vi "Main.vi"() -> ()   [LabVIEW 2021]
doc: "Use this template to build a simple state machine design pattern. Each state executes code and determines which state to transition to."
uses:
  controls/State.ctl
  controls/Data.ctl
  vmmso/vmmso.lvlib
panel:
  out "IO Read Return":u32 format="%x"
  out "IO4":bool
  out "IO0":bool
  out "Is IO Ready?":bool
  in  "DDS2 Amplitude":dbl=2000.0
  in  "DDS2 Bias":dbl
  in  "DDS2 Freq":dbl=1000.0
  in  "DDS2 Wave Style":u16(ring) items=["Sine", "Square", "Ramp"]
  in  "DDS1 Amplitude":dbl=2000.0
  in  "DDS1 Bias":dbl
  in  "DDS1 Freq":dbl=1000.0
  in  "DDS1 Wave Style":u16(ring) items=["Sine", "Square", "Ramp"]
  out "Is Data Ready？":bool
  out "ReadVoltageData Return":u32
  out "Voltage Wave":dbl[][](graph)
  out "Capture Return":i32
  out "Device is OK?":bool
  out "Support Samples":u32[](array[numeric])
  in  "Exit":bool
  # "DDS1"
  # "DDS2"
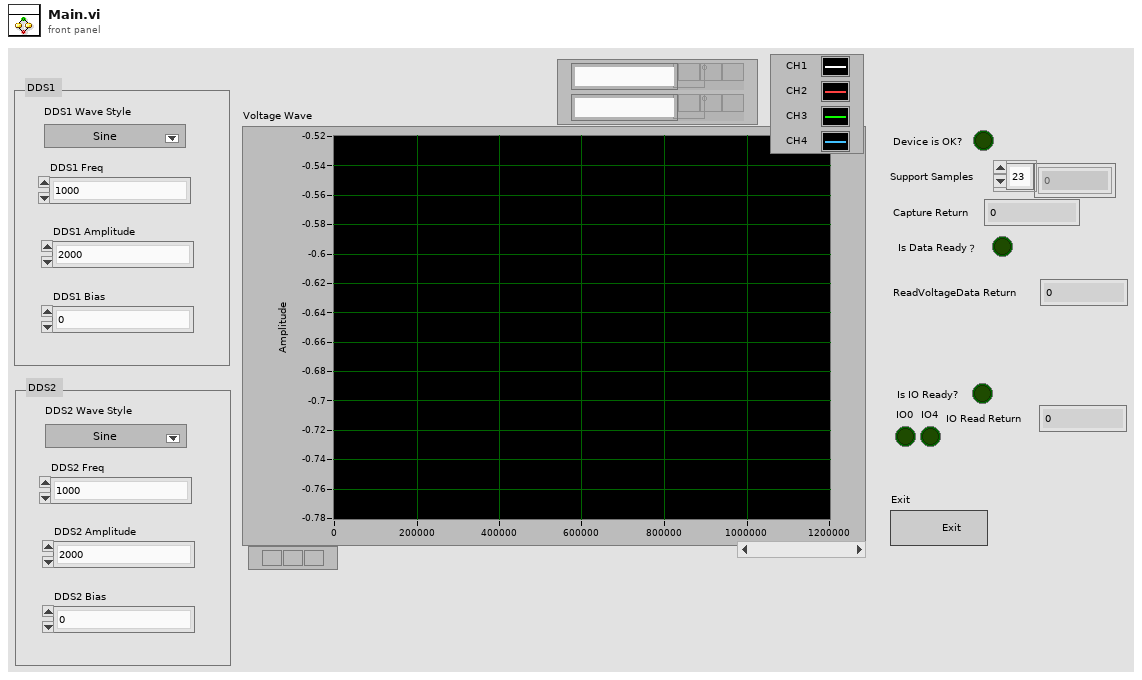
[diagram p1: front panel]
types:
  T1 = typedef "Data.ctl" = cluster{"Boolean <Is Exit>":bool, "String <Replace Me>":string, "Numeric <Replace Me>":dbl}
  T2 = typedef "State.ctl" = enum16{"Initialize", "Wait for UsbIn", "Init Osc and Dds", "Wait for Event", "Capture", "Read Voltage", "Read IO", "Exit"}
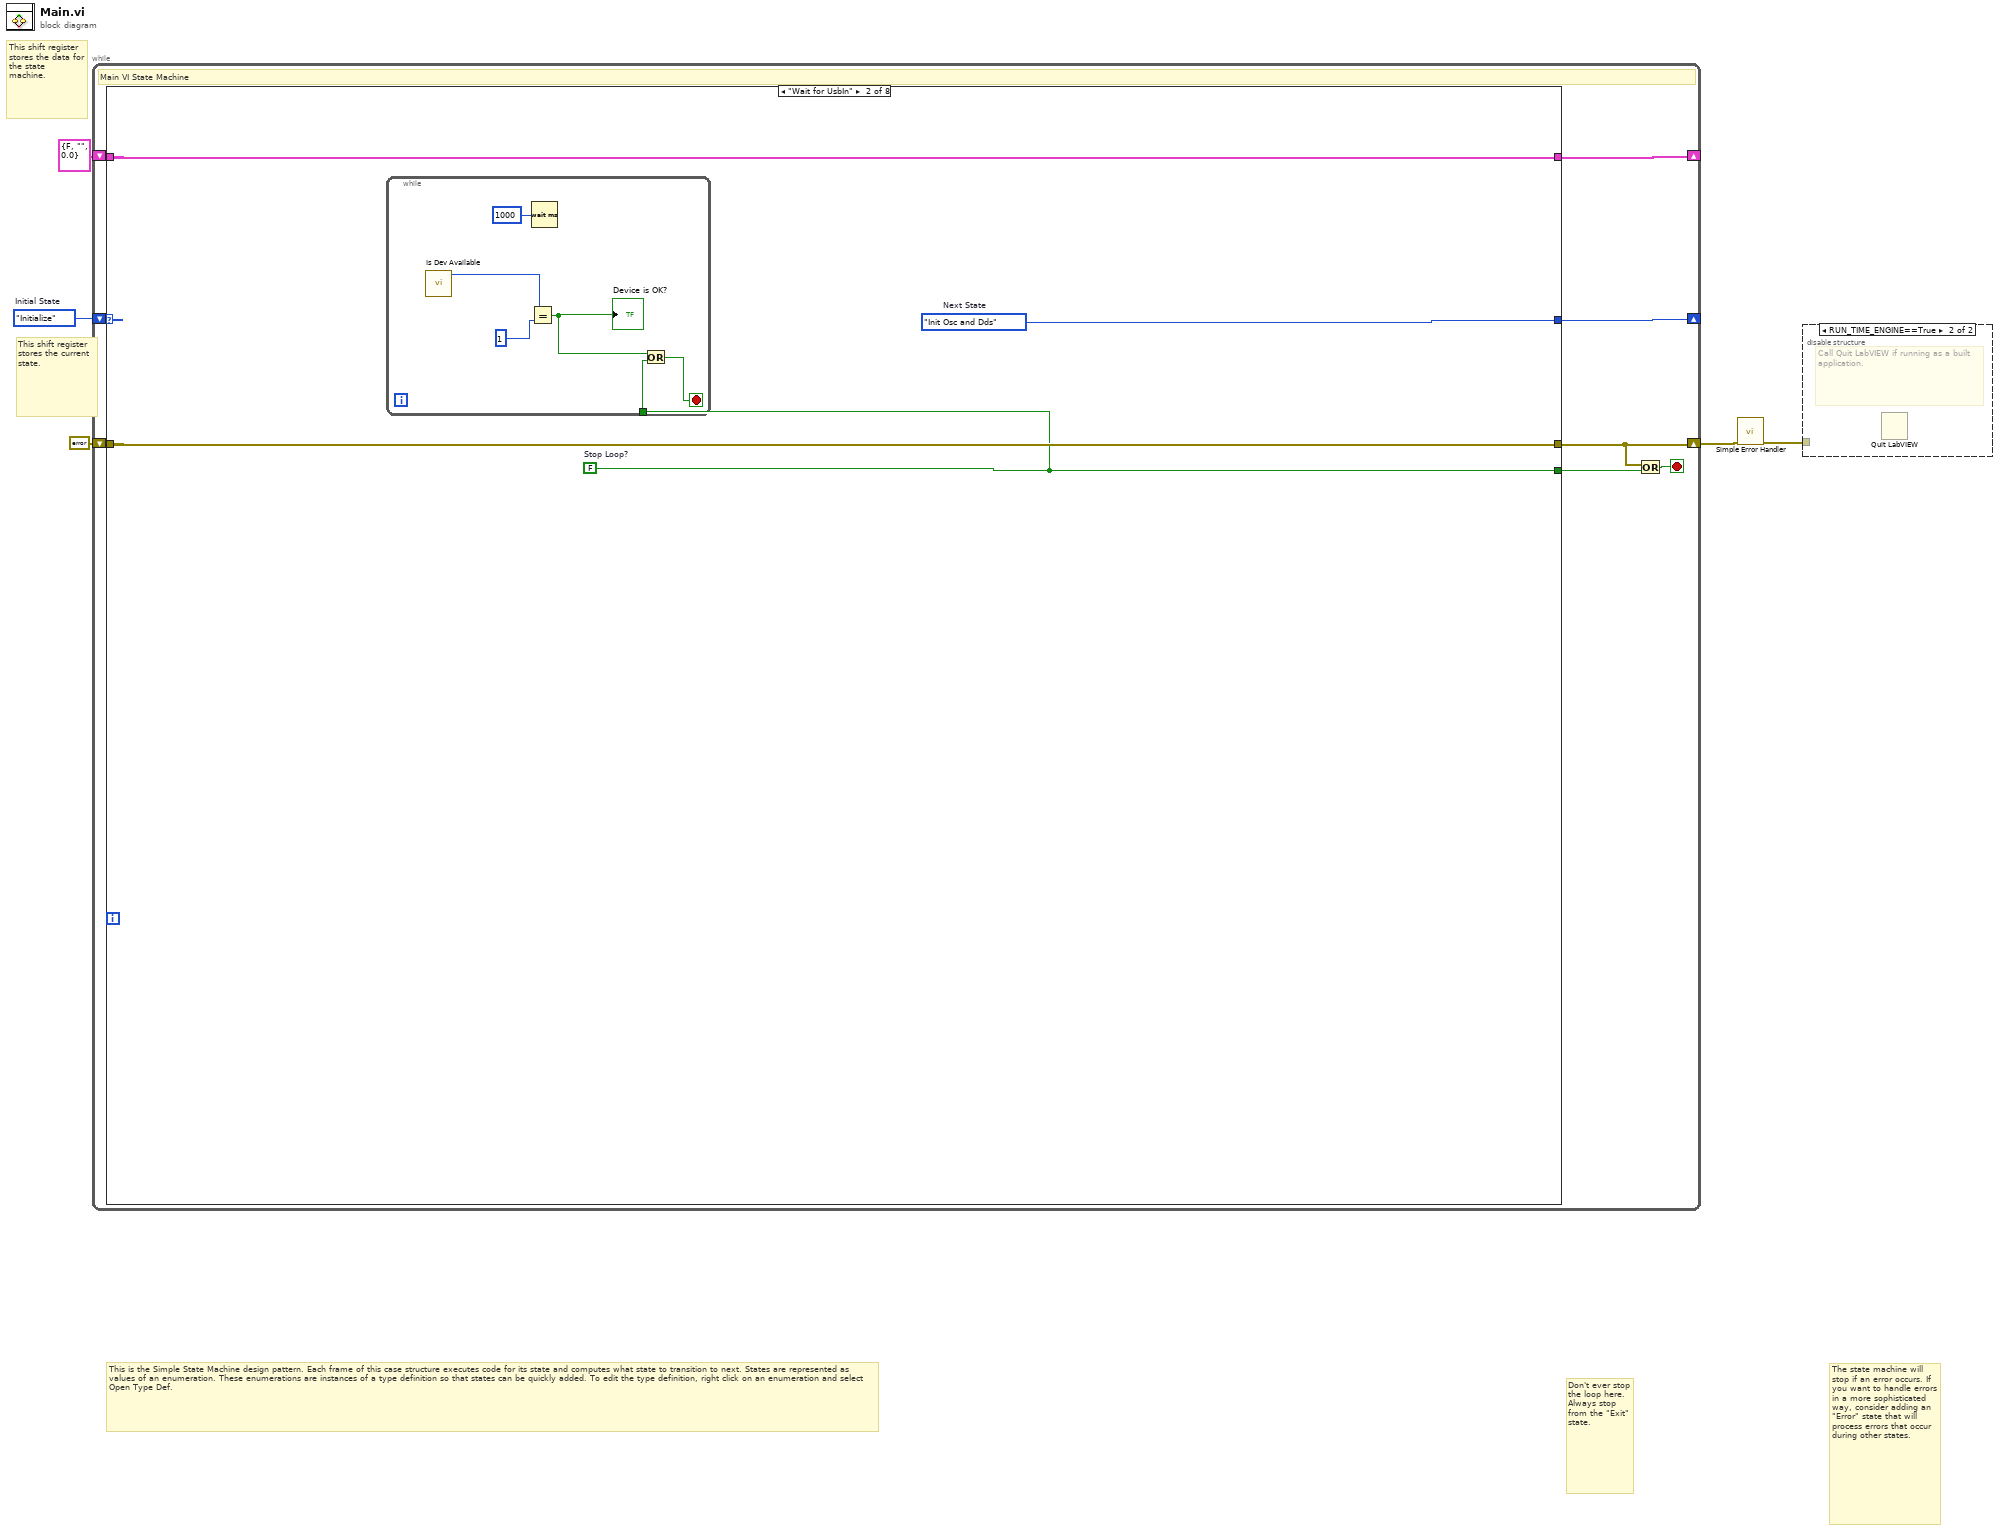
[diagram p0: block diagram]
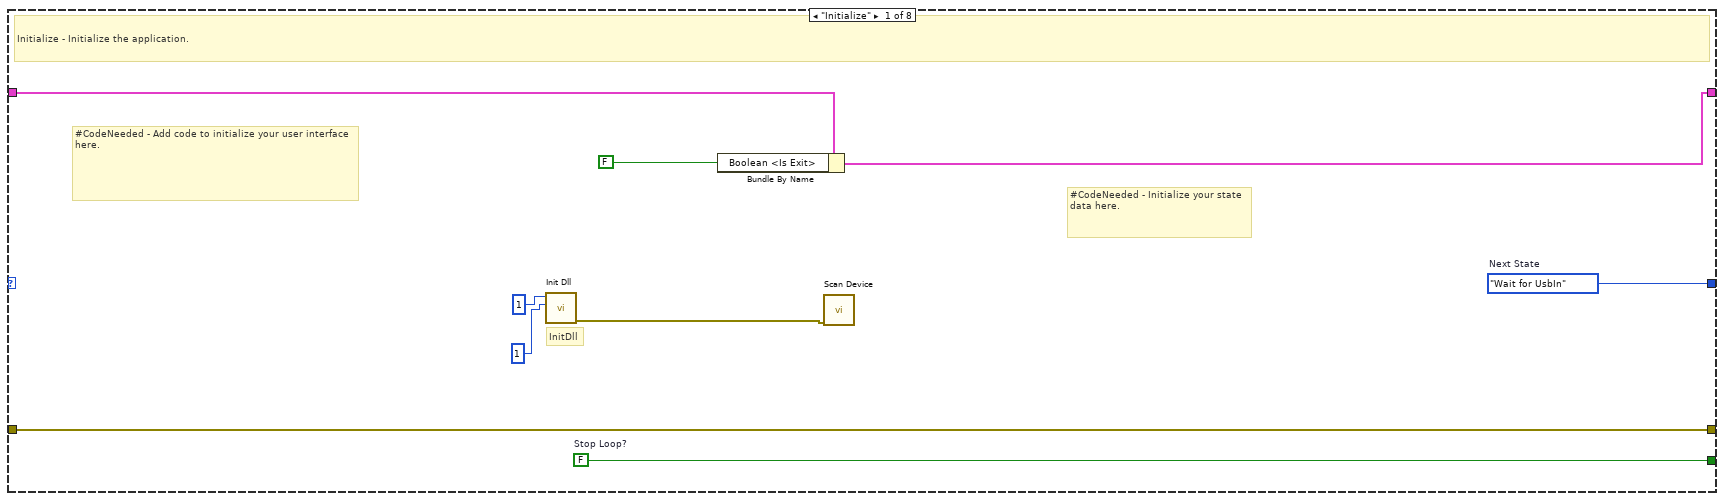
[diagram p3: hidden frame]
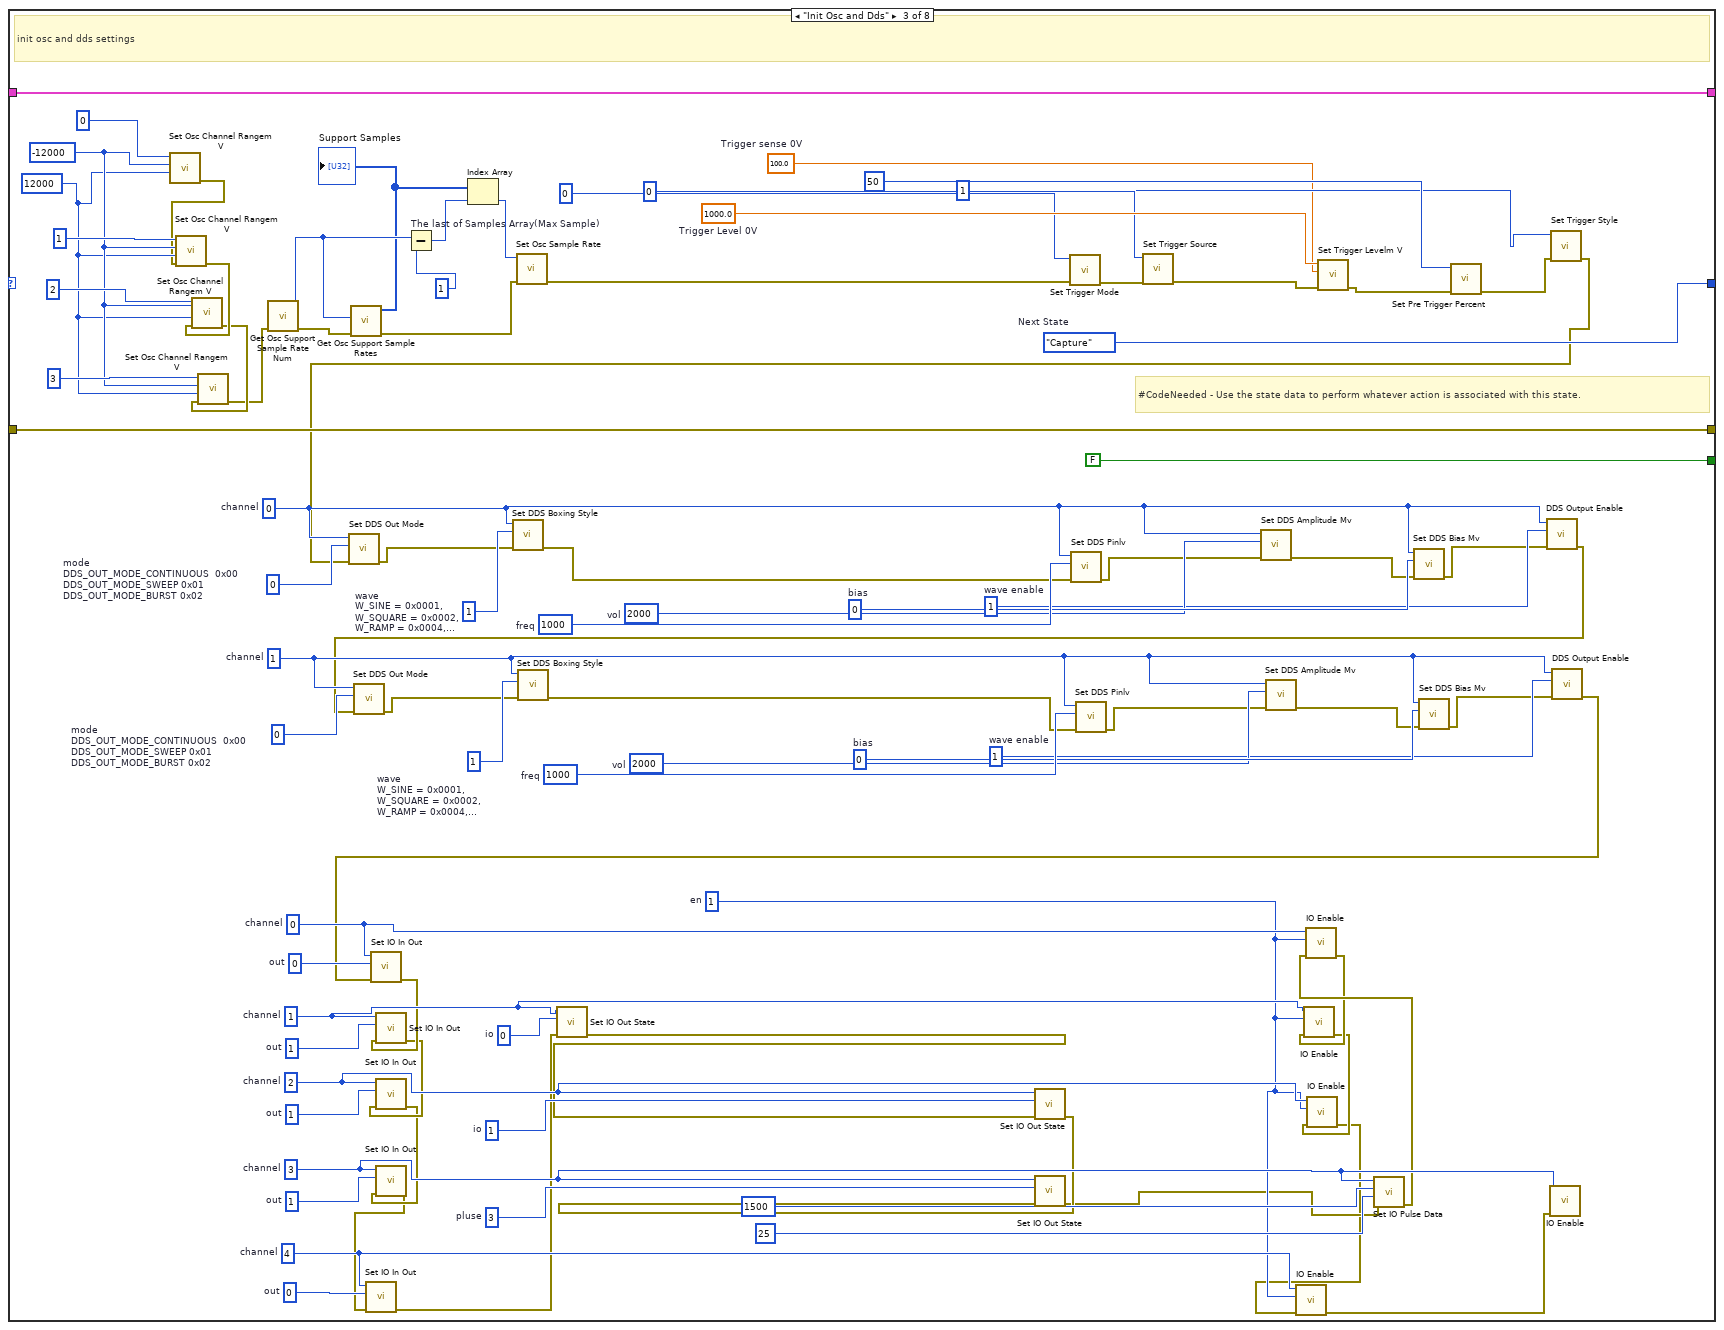
[diagram p4: hidden frame]
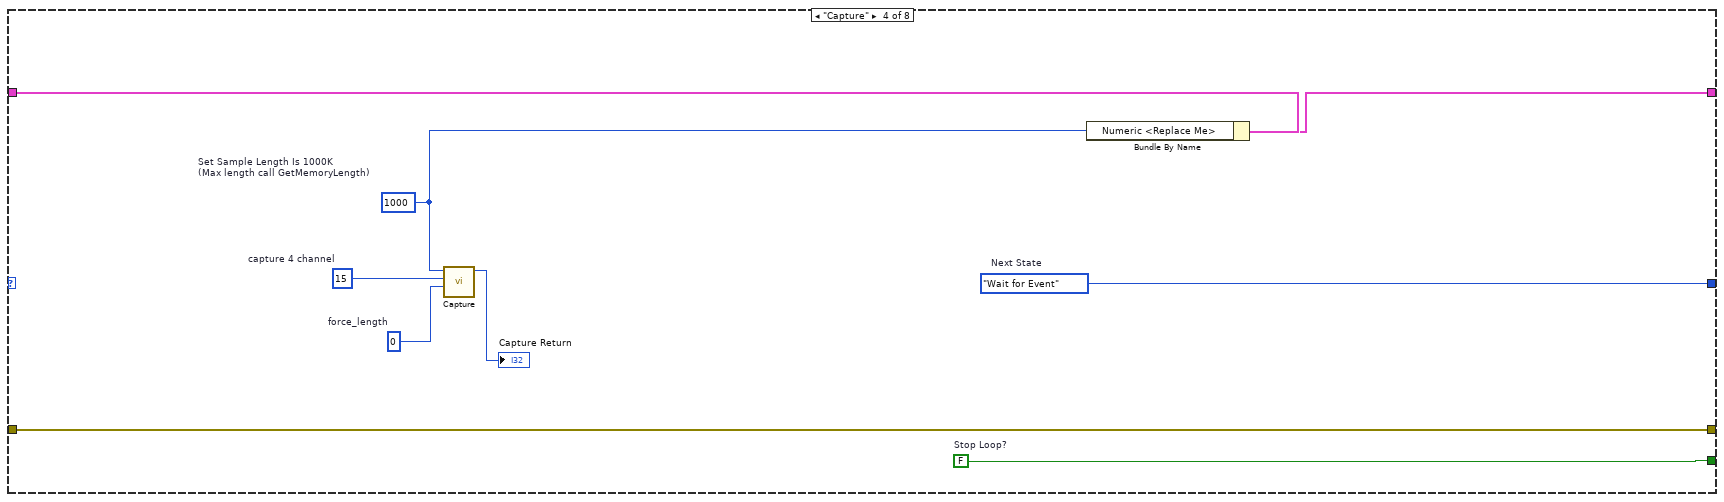
[diagram p5: hidden frame]
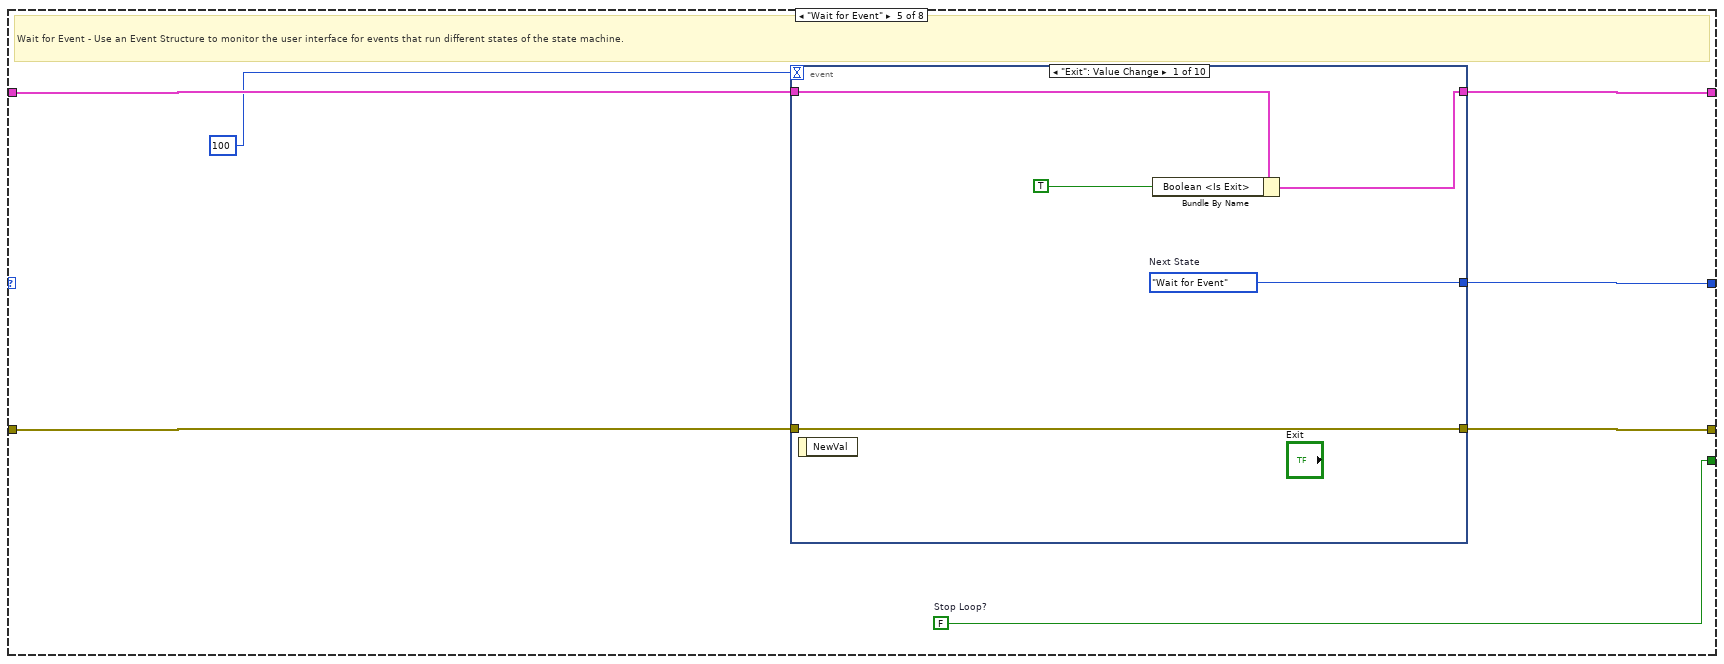
[diagram p6: hidden frame]
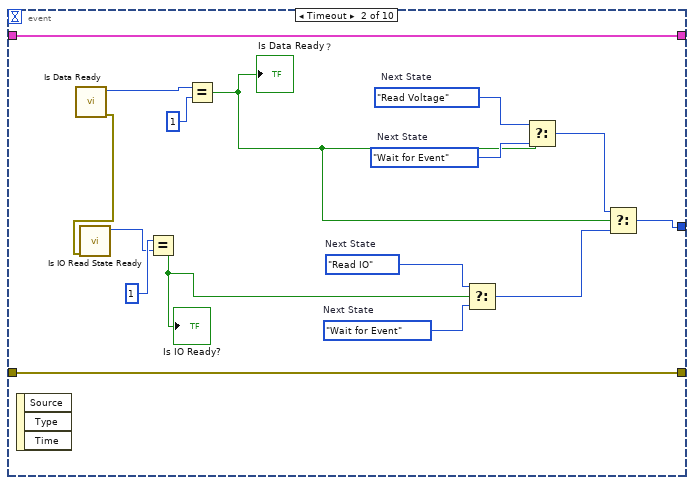
[diagram p7: hidden frame]
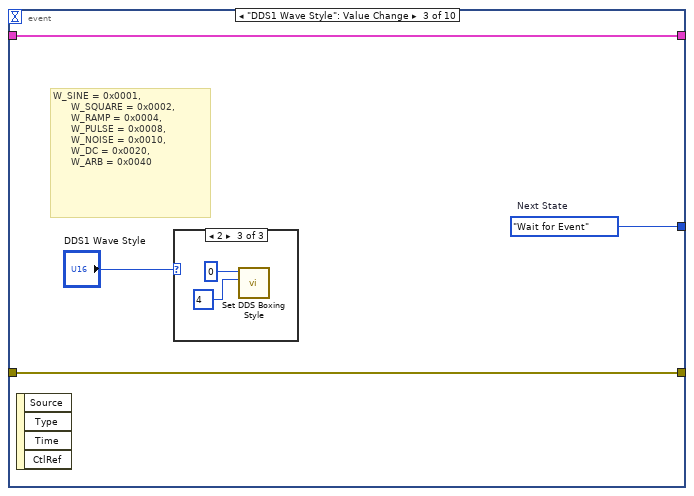
[diagram p8: hidden frame]
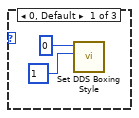
[diagram p9: hidden frame]
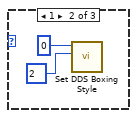
[diagram p10: hidden frame]
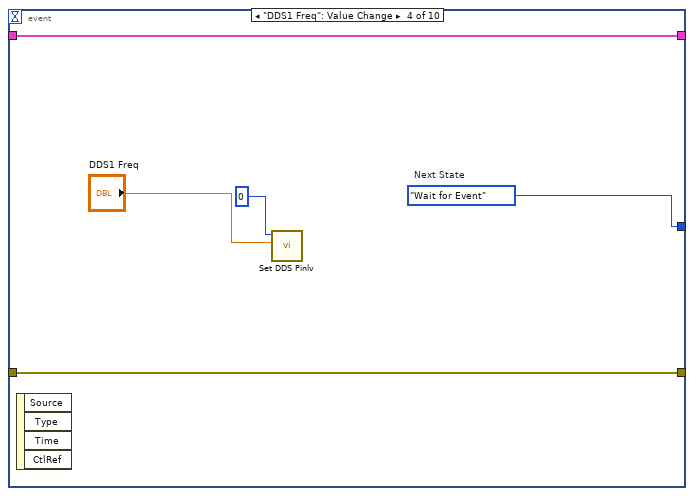
[diagram p11: hidden frame]
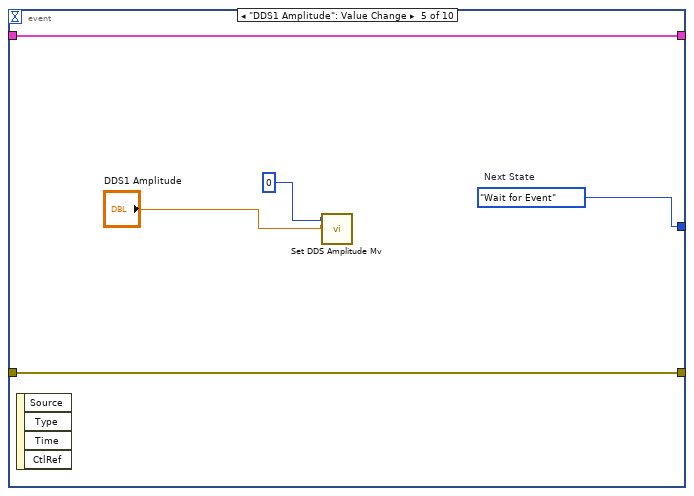
[diagram p12: hidden frame]
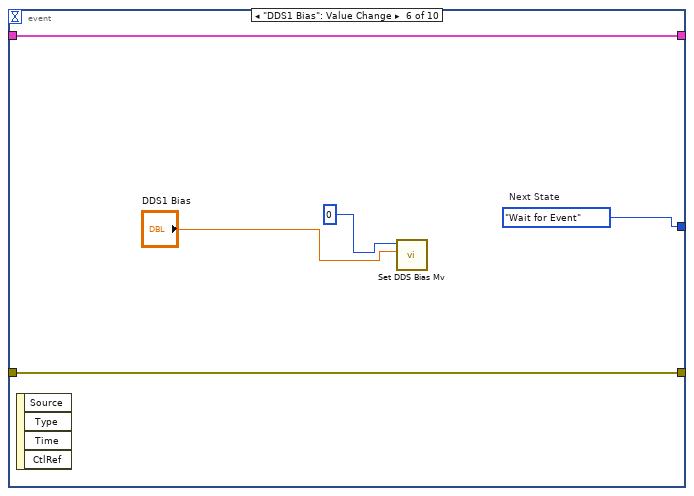
[diagram p13: hidden frame]
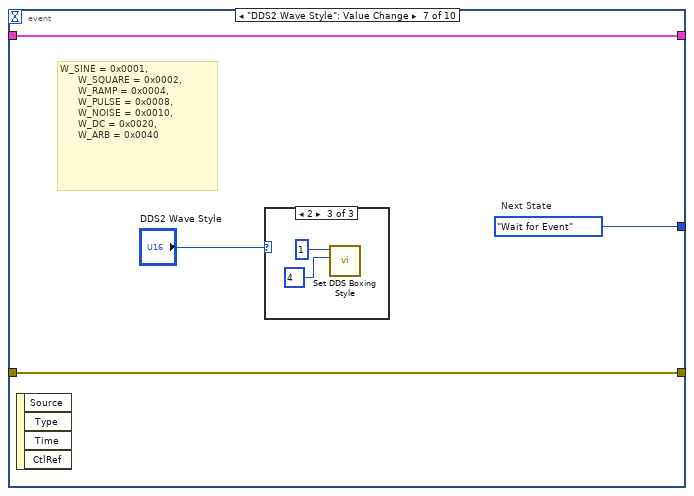
[diagram p14: hidden frame]
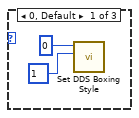
[diagram p15: hidden frame]
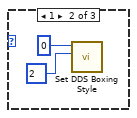
[diagram p16: hidden frame]
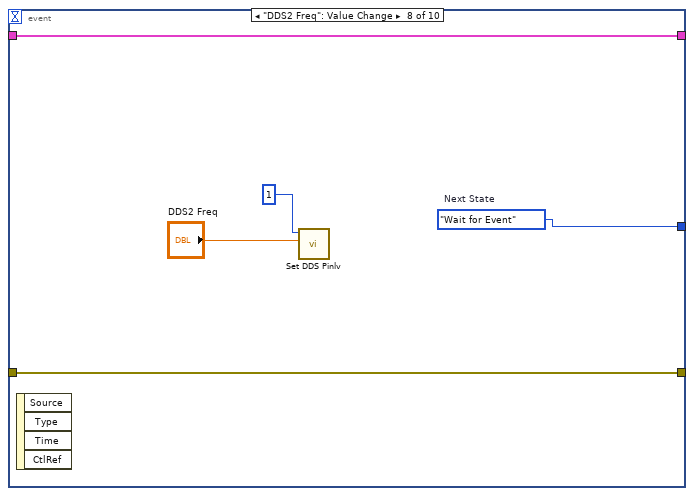
[diagram p17: hidden frame]
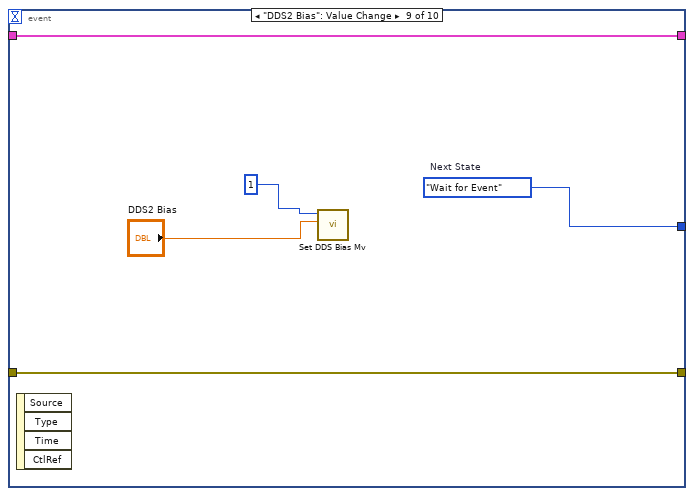
[diagram p18: hidden frame]
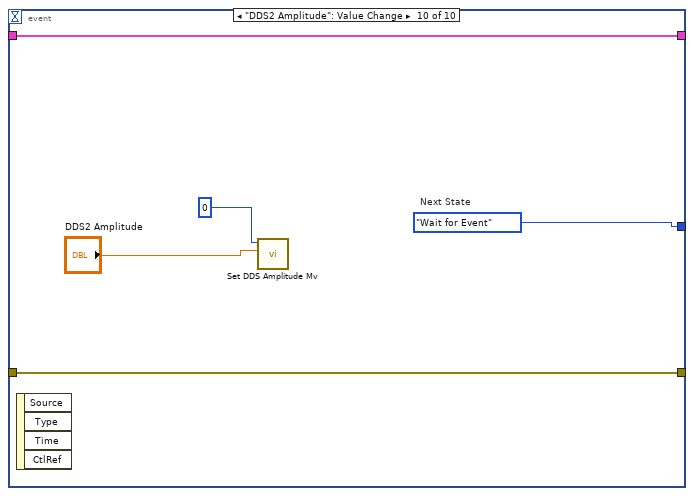
[diagram p19: hidden frame]
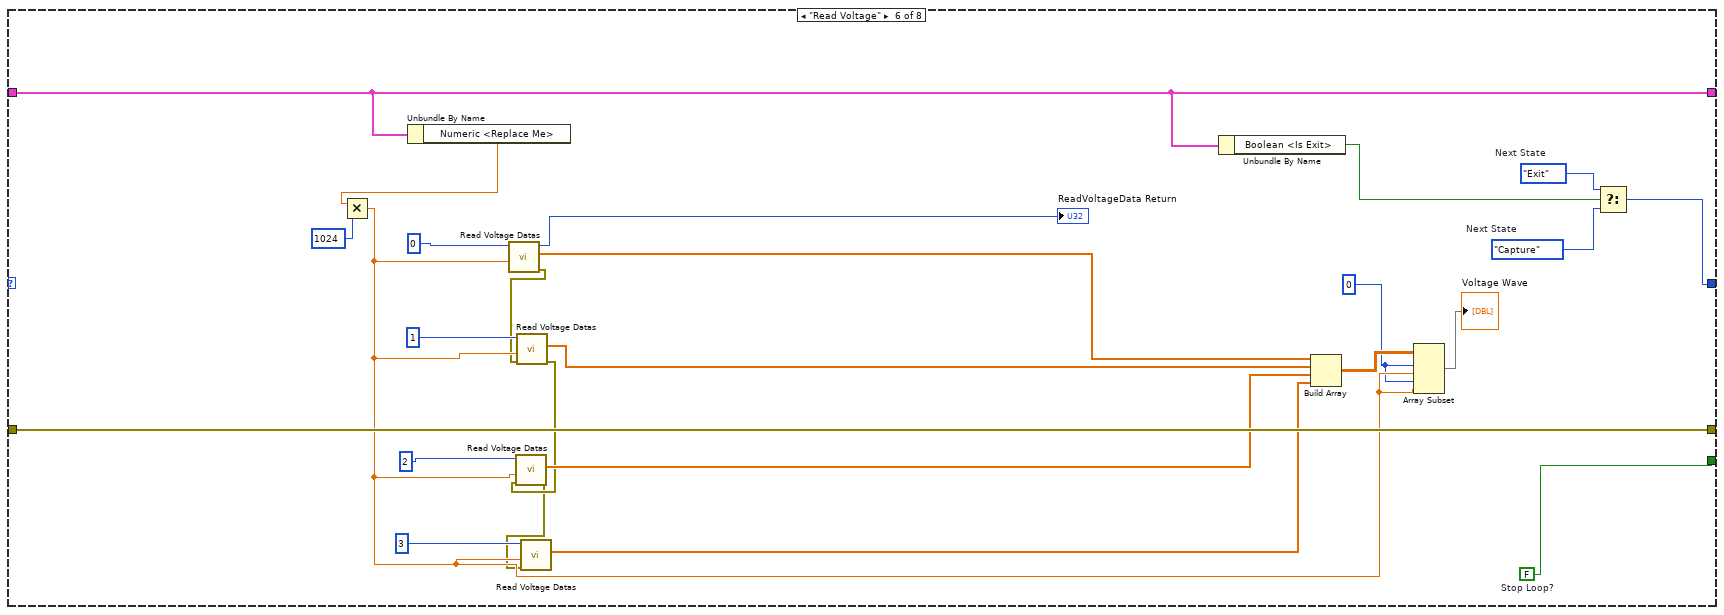
[diagram p20: hidden frame]
diagram:
  w5 = State."Initialize"  # Initial State
  # "Don't ever stop the loop here. Always stop from the \"Exit\" state."
  # "The state machine will stop if an error occurs. If you want to handle errors in a more sophisticated way, consider adding an \"Error\" state that will process errors that occur during other states."
  # "This shift register stores the data for the state machine."
  # "This is the Simple State Machine design pattern. Each frame of this case structure executes code for its state and computes what state to transition to next. States are represented as values of an enumeration. These enumerations are instances of a type definition so that states can be quickly added. To edit the type definition, right click on an enumeration and select Open Type Def."
  # "This shift register stores the current state."
  n1 = while {
    shift-right: [w12] -> _
    shift-left: w5 -> [w13]
    shift-right: [w10] -> _
    shift-left: T1 {"Boolean <Is Exit>"=FALSE, "String <Replace Me>"="", "Numeric <Replace Me>"=0.0} ("Data") -> [w11]
    shift-right: [w7] -> w2
    shift-left: errorcluster {"status"=FALSE, "code"=0, "source"=""} ("error constant") -> [w9]
    stop <- w8 stop-if-true
    # "Main VI State Machine"
    n2 = case shown="\"Wait for UsbIn\"" w13 {
      tunnel: [w22 w25 w120 w128 w136 w209 w234 w248] -> w12
      tunnel: w11 -> [w15 w23 w118 w123 w135 w212 w243 w247]
      tunnel: [w14 w23 w118 w122 w134 w212 w243 w247] -> w10
      tunnel: w9 -> [w20 w26 w117 w129 w133 w232 w242 w245]
      tunnel: [w20 w26 w117 w129 w132 w232 w242 w245] -> w7
      tunnel: [w21 w24 FALSE ("Stop Loop?") w127 w130 w231 w233 w246] -> w6
      frame "Initialize" {
        w21 = FALSE  # Stop Loop?
        w22 = State."Wait for UsbIn"  # Next State
        # "InitDll"
        # "#CodeNeeded - Initialize your state data here."
        # "#CodeNeeded - Add code to initialize your user interface here."
        # "Initialize - Initialize the application."
        n3 = call "Init Dll.vi"("en_hard_watchdog"=1 ("channel"), "en_log"=1 ("channel")) -> ("error out"=w17:errorcluster)  [unwired: 8 in, 1 out]
        n4 = Bundle By Name(cluster=w15, "Boolean <Is Exit>"=FALSE) -> (w14:T1)
        n5 = call "Scan Device.vi"("error in (no error)"=w17) -> ()  [unwired: 9 in, 2 out]
      }
      frame "Wait for UsbIn" {
        w25 = State."Init Osc and Dds"  # Next State
        w24 = FALSE  # Stop Loop?
        n6 = while {
          tunnel: w24 -> [w30]
          stop <- w29 stop-if-true
          n7 = call "Is Dev Available.vi"() -> ("function return"=w28:i32)  [unwired: 10 in, 1 out]
          n8 = Equal?(x=w28, y=1 ("channel")) -> (x = y?=w27:bool)
          "Device is OK?" <- w27
          n9 = Wait (ms)(milliseconds to wait=u32 1000 ("等待时间（毫秒）")) -> ()  [unwired: 1 out]
          n10 = Or(x=w27, y=w30) -> (x .or. y?=w29:bool)
        }
      }
      frame "Init Osc and Dds" {
        w72 = i8 0  # out
        w71 = i8 4  # channel
        w76 = i8 3  # pluse
        w77 = i8 1  # out
        w75 = i8 3  # channel
        w70 = i8 1  # en
        w81 = i8 0  # io
        w82 = i8 1  # io
        w83 = i8 1  # out
        w78 = i8 2  # channel
        w84 = i8 1  # out
        w79 = i8 1  # channel
        w85 = i8 0  # out
        w80 = i8 0  # channel
        w86 = sgl 100.0  # Trigger sense 0V
        w93 = i8 0  # mode DDS_OUT_MODE_CONTINUOUS  0x00 DDS_OUT_MODE_SWEEP 0x01 DDS_OUT_MODE_BURST 0x02
        w95 = i8 1  # wave enable
        w97 = u32 0  # bias
        w96 = u32 2000  # vol
        w98 = u32 1000  # freq
        w99 = i8 1  # wave  W_SINE = 0x0001,  W_SQUARE = 0x0002,  W_RAMP = 0x0004,  W_PULSE = 0x0008,  W_NOISE = 0x0010,  W_DC = 0x0020,  W_ARB = 0x0040
        w94 = i8 1  # channel
        w100 = i8 0  # mode DDS_OUT_MODE_CONTINUOUS  0x00 DDS_OUT_MODE_SWEEP 0x01 DDS_OUT_MODE_BURST 0x02
        w102 = i8 1  # wave enable
        w104 = u32 0  # bias
        w103 = u32 2000  # vol
        w105 = u32 1000  # freq
        w106 = i8 1  # wave  W_SINE = 0x0001,  W_SQUARE = 0x0002,  W_RAMP = 0x0004,  W_PULSE = 0x0008,  W_NOISE = 0x0010,  W_DC = 0x0020,  W_ARB = 0x0040
        w101 = i8 0  # channel
        w114 = sgl 1000.0  # Trigger Level 0V
        w88 = 12000 ("minmv")
        w89 = -12000 ("minmv")
        w120 = State."Capture"  # Next State
        # "#CodeNeeded - Use the state data to perform whatever action is associated with this state."
        # "init osc and dds settings"
        n11 = call "Set Osc Channel Rangem V.vi"("maxmv"=w88, "minmv"=w89, "channel"=0) -> ("error out"=w69:errorcluster)  [unwired: 7 in, 1 out]
        n12 = call "Set Osc Channel Rangem V.vi"("error in (no error)"=w69, "maxmv"=w88, "minmv"=w89, "channel"=1) -> ("error out"=w68:errorcluster)  [unwired: 6 in, 1 out]
        n13 = call "Set Osc Channel Rangem V.vi"("error in (no error)"=w68, "maxmv"=w88, "minmv"=w89, "channel"=2) -> ("error out"=w67:errorcluster)  [unwired: 6 in, 1 out]
        n14 = call "Set Osc Channel Rangem V.vi"("error in (no error)"=w67, "maxmv"=w88, "minmv"=w89, "channel"=3) -> ("error out"=w66:errorcluster)  [unwired: 6 in, 1 out]
        n15 = call "Get Osc Support Sample Rate Num.vi"("error in (no error)"=w66) -> ("error out"=w65:errorcluster, "function return"=w111:i32)  [unwired: 9 in]
        n16 = call "Get Osc Support Sample Rates.vi"("error in (no error)"=w65, "maxnum"=w111) -> ("error out"=w64:errorcluster, "sample out"=w108:u32[])  [unwired: 7 in, 1 out]
        "Support Samples" <- w108
        n17 = Subtract "The last of Samples Array(Max Sample)"(x=w111, y=1 ("front")) -> (x-y=w113:i32)
        n18 = Index Array(array=w108, index=w113) -> (element=w87:u32)
        n19 = call "Set Osc Sample Rate.vi"("error in (no error)"=w64, "sample"=w87) -> ("error out"=w63:errorcluster)  [unwired: 8 in, 1 out]
        n20 = call "Set Trigger Mode.vi"("error in (no error)"=w63, "mode"=0 ("front")) -> ("error out"=w62:errorcluster)  [unwired: 9 in]
        n21 = call "Set Trigger Source.vi"("error in (no error)"=w62, "source"=0 ("front")) -> ("error out"=w61:errorcluster)  [unwired: 9 in]
        n22 = call "Set Trigger Levelm V.vi"("error in (no error)"=w61, "sense_mv"=w86, "level_mv"=w114) -> ("error out"=w60:errorcluster)  [unwired: 8 in]
        n23 = call "Set Pre Trigger Percent.vi"("error in (no error)"=w60, "front"=50) -> ("error out"=w59:errorcluster)  [unwired: 9 in]
        n24 = call "Set Trigger Style.vi"("error in (no error)"=w59, "style"=u32 1) -> ("error out"=w58:errorcluster)  [unwired: 9 in]
        n25 = call "Set DDS Out Mode.vi"("error in (no error)"=w58, "out_mode"=w100, "channel_index"=w101) -> ("error out"=w57:errorcluster)  [unwired: 8 in]
        n26 = call "Set DDS Boxing Style.vi"("error in (no error)"=w57, "boxing"=w106, "channel_index"=w101) -> ("error out"=w56:errorcluster)  [unwired: 8 in]
        n27 = call "Set DDS Pinlv.vi"("error in (no error)"=w56, "pinlv"=w105, "channel_index"=w101) -> ("error out"=w55:errorcluster)  [unwired: 8 in]
        n28 = call "Set DDS Amplitude Mv.vi"("error in (no error)"=w55, "amplitdude"=w103, "channel_index"=w101) -> ("error out"=w54:errorcluster)  [unwired: 8 in]
        n29 = call "Set DDS Bias Mv.vi"("error in (no error)"=w54, "bias"=w104, "channel_index"=w101) -> ("error out"=w53:errorcluster)  [unwired: 8 in]
        n30 = call "DDS Output Enable.vi"("error in (no error)"=w53, "enable"=w102, "channel_index"=w101) -> ("error out"=w52:errorcluster)  [unwired: 8 in]
        n31 = call "Set DDS Out Mode.vi"("error in (no error)"=w52, "out_mode"=w93, "channel_index"=w94) -> ("error out"=w51:errorcluster)  [unwired: 8 in]
        n32 = call "Set DDS Boxing Style.vi"("error in (no error)"=w51, "boxing"=w99, "channel_index"=w94) -> ("error out"=w50:errorcluster)  [unwired: 8 in]
        n33 = call "Set DDS Pinlv.vi"("error in (no error)"=w50, "pinlv"=w98, "channel_index"=w94) -> ("error out"=w49:errorcluster)  [unwired: 8 in]
        n34 = call "Set DDS Amplitude Mv.vi"("error in (no error)"=w49, "amplitdude"=w96, "channel_index"=w94) -> ("error out"=w48:errorcluster)  [unwired: 8 in]
        n35 = call "Set DDS Bias Mv.vi"("error in (no error)"=w48, "bias"=w97, "channel_index"=w94) -> ("error out"=w47:errorcluster)  [unwired: 8 in]
        n36 = call "DDS Output Enable.vi"("error in (no error)"=w47, "enable"=w95, "channel_index"=w94) -> ("error out"=w46:errorcluster)  [unwired: 8 in]
        n37 = call "Set IO In Out.vi"("error in (no error)"=w46, "inout"=w85, "channel"=w80) -> ("error out"=w45:errorcluster)  [unwired: 8 in]
        n38 = call "Set IO In Out.vi"("error in (no error)"=w45, "inout"=w84, "channel"=w79) -> ("error out"=w44:errorcluster)  [unwired: 8 in]
        n39 = call "Set IO In Out.vi"("error in (no error)"=w44, "inout"=w83, "channel"=w78) -> ("error out"=w43:errorcluster)  [unwired: 8 in]
        n40 = call "Set IO In Out.vi"("error in (no error)"=w43, "inout"=w77, "channel"=w75) -> ("error out"=w42:errorcluster)  [unwired: 8 in]
        n41 = call "Set IO In Out.vi"("error in (no error)"=w42, "inout"=w72, "channel"=w71) -> ("error out"=w41:errorcluster)  [unwired: 8 in]
        n42 = call "Set IO Out State.vi"("error in (no error)"=w41, "state"=w81, "channel"=w79) -> ("error out"=w40:errorcluster)  [unwired: 8 in]
        n43 = call "Set IO Out State.vi"("error in (no error)"=w40, "state"=w82, "channel"=w78) -> ("error out"=w39:errorcluster)  [unwired: 8 in]
        n44 = call "Set IO Out State.vi"("error in (no error)"=w39, "state"=w76, "channel"=w75) -> ("error out"=w38:errorcluster)  [unwired: 8 in]
        n45 = call "Set IO Pulse Data.vi"("error in (no error)"=w38, "duty"=25 ("minmv"), "hz"=1500 ("minmv"), "channel"=w75) -> ("error out"=w37:errorcluster)  [unwired: 7 in]
        n46 = call "IO Enable.vi"("error in (no error)"=w37, "enable"=w70, "channel"=w80) -> ("error out"=w36:errorcluster)  [unwired: 8 in]
        n47 = call "IO Enable.vi"("error in (no error)"=w36, "enable"=w70, "channel"=w79) -> ("error out"=w35:errorcluster)  [unwired: 8 in]
        n48 = call "IO Enable.vi"("error in (no error)"=w35, "enable"=w70, "channel"=w78) -> ("error out"=w34:errorcluster)  [unwired: 8 in]
        n49 = call "IO Enable.vi"("error in (no error)"=w34, "enable"=w70, "channel"=w71) -> ("error out"=w33:errorcluster)  [unwired: 8 in]
        n50 = call "IO Enable.vi"("error in (no error)"=w33, "channel"=w75) -> ()  [unwired: 9 in, 1 out]
      }
      frame "Capture" {
        w124 = i8 0  # force_length
        w121 = u32 1000  # Set Sample Length Is 1000K (Max length call GetMemoryLength)
        w125 = i8 15  # capture 4 channel
        w127 = FALSE  # Stop Loop?
        w128 = State."Wait for Event"  # Next State
        n51 = call "Capture.vi"("force_length"=w124, "capture_channel"=w125, "length"=w121) -> ("function return"=→"Capture Return":i32)  [unwired: 7 in, 1 out]
        n52 = Bundle By Name(cluster=w123, "Numeric <Replace Me>"=w121) -> (w122:T1)
      }
      frame "Wait for Event" {
        w130 = FALSE  # Stop Loop?
        # "Wait for Event - Use an Event Structure to monitor the user interface for events that run different states of the state machine."
        n53 = event shown="[0] \"Exit\": Value Change" {
          selector: _ -> [_ _ _ _ _ _ _ _ _ _]
          dyn-events: _ -> [_ _ _ _ _ _ _ _ _ _]
          timeout: 100 ("y") -> [_ _ _ _ _ _ _ _ _ _]
          tunnel: [w141 w144 w158 w170 w175 w180 w184 w194 w199 w204] -> w136
          tunnel: w135 -> [w138 w157 w161 w172 w177 w182 w186 w197 w202 w207]
          tunnel: [w137 w157 w161 w172 w177 w182 w186 w197 w202 w207] -> w134
          tunnel: w133 -> [w140 w156 w160 w171 w176 w181 w185 w196 w201 w206]
          tunnel: [w140 w156 w160 w171 w176 w181 w185 w196 w201 w206] -> w132
          event "Exit": Value Change {
            w141 = State."Wait for Event"  # Next State
            n54 = event-data() -> ()  [unwired: 1 in, 1 out]
            n55 = Bundle By Name(cluster=w138, "Boolean <Is Exit>"=TRUE) -> (w137:T1)
          }
          event Timeout {
            w149 = State."Wait for Event"  # Next State
            w150 = State."Read IO"  # Next State
            w152 = State."Wait for Event"  # Next State
            w153 = State."Read Voltage"  # Next State
            n56 = event-data() -> ()  [unwired: 1 in, 3 out]
            n57 = call "Is Data Ready.vi"() -> ("error out"=w142:errorcluster, "function return"=w155:i32)  [unwired: 10 in]
            n58 = call "Is IO Read State Ready.vi"("error in (no error)"=w142) -> ("function return"=w143:i32)  [unwired: 9 in, 1 out]
            n59 = Equal?(x=1 ("y"), y=w143) -> (x = y?=w151:bool)
            "Is IO Ready?" <- w151
            n60 = Equal?(x=w155, y=1) -> (x = y?=w145:bool)
            "Is Data Ready？" <- w145
            n61 = Select(t=w150, s=w151, f=w149) -> (s? t:f=w147:T2)
            n62 = Select(t=w153, s=w145, f=w152) -> (s? t:f=w146:T2)
            n63 = Select(t=w146, s=w145, f=w147) -> (s? t:f=w144:T2)
          }
          event "DDS1 Wave Style": Value Change {
            w158 = State."Wait for Event"  # Next State
            # "W_SINE = 0x0001, \n\t\t\t\t\t\tW_SQUARE = 0x0002, \n\t\t\t\t\t\tW_RAMP = 0x0004, \n\t\t\t\t\t\tW_PULSE = 0x0008, \n\t\t\t\t\t\tW_NOISE = 0x0010, \n\t\t\t\t\t\tW_DC = 0x0020, \n\t\t\t\t\t\tW_ARB = 0x0040"
            n64 = event-data() -> ()  [unwired: 1 in, 4 out]
            n65 = case shown="2" "DDS1 Wave Style" {
              frame 0, Default {
                n66 = call "Set DDS Boxing Style.vi"("boxing"=1 ("y"), "channel_index"=0 ("y")) -> ()  [unwired: 9 in, 1 out]
              }
              frame 1 {
                n67 = call "Set DDS Boxing Style.vi"("boxing"=2 ("y"), "channel_index"=0 ("y")) -> ()  [unwired: 9 in, 1 out]
              }
              frame 2 {
                n68 = call "Set DDS Boxing Style.vi"("boxing"=4 ("y"), "channel_index"=0 ("y")) -> ()  [unwired: 9 in, 1 out]
              }
            }
          }
          event "DDS1 Freq": Value Change {
            w170 = State."Wait for Event"  # Next State
            n69 = event-data() -> ()  [unwired: 1 in, 4 out]
            n70 = call "Set DDS Pinlv.vi"("pinlv"="DDS1 Freq", "channel_index"=0 ("y")) -> ()  [unwired: 9 in, 1 out]
          }
          event "DDS1 Amplitude": Value Change {
            w175 = State."Wait for Event"  # Next State
            n71 = event-data() -> ()  [unwired: 1 in, 4 out]
            n72 = call "Set DDS Amplitude Mv.vi"("amplitdude"="DDS1 Amplitude", "channel_index"=0 ("y")) -> ()  [unwired: 9 in, 1 out]
          }
          event "DDS1 Bias": Value Change {
            w180 = State."Wait for Event"  # Next State
            n73 = event-data() -> ()  [unwired: 1 in, 4 out]
            n74 = call "Set DDS Bias Mv.vi"("bias"="DDS1 Bias", "channel_index"=0 ("y")) -> ()  [unwired: 9 in, 1 out]
          }
          event "DDS2 Wave Style": Value Change {
            w184 = State."Wait for Event"  # Next State
            # "W_SINE = 0x0001, \n\t\t\t\t\t\tW_SQUARE = 0x0002, \n\t\t\t\t\t\tW_RAMP = 0x0004, \n\t\t\t\t\t\tW_PULSE = 0x0008, \n\t\t\t\t\t\tW_NOISE = 0x0010, \n\t\t\t\t\t\tW_DC = 0x0020, \n\t\t\t\t\t\tW_ARB = 0x0040"
            n75 = event-data() -> ()  [unwired: 1 in, 4 out]
            n76 = case shown="2" "DDS2 Wave Style" {
              frame 0, Default {
                n77 = call "Set DDS Boxing Style.vi"("boxing"=1 ("y"), "channel_index"=0 ("y")) -> ()  [unwired: 9 in, 1 out]
              }
              frame 1 {
                n78 = call "Set DDS Boxing Style.vi"("boxing"=2 ("y"), "channel_index"=0 ("y")) -> ()  [unwired: 9 in, 1 out]
              }
              frame 2 {
                n79 = call "Set DDS Boxing Style.vi"("boxing"=4 ("y"), "channel_index"=1 ("y")) -> ()  [unwired: 9 in, 1 out]
              }
            }
          }
          event "DDS2 Freq": Value Change {
            w194 = State."Wait for Event"  # Next State
            n80 = event-data() -> ()  [unwired: 1 in, 4 out]
            n81 = call "Set DDS Pinlv.vi"("pinlv"="DDS2 Freq", "channel_index"=1 ("y")) -> ()  [unwired: 9 in, 1 out]
          }
          event "DDS2 Bias": Value Change {
            w199 = State."Wait for Event"  # Next State
            n82 = event-data() -> ()  [unwired: 1 in, 4 out]
            n83 = call "Set DDS Bias Mv.vi"("bias"="DDS2 Bias", "channel_index"=1 ("y")) -> ()  [unwired: 9 in, 1 out]
          }
          event "DDS2 Amplitude": Value Change {
            w204 = State."Wait for Event"  # Next State
            n84 = event-data() -> ()  [unwired: 1 in, 4 out]
            n85 = call "Set DDS Amplitude Mv.vi"("amplitdude"="DDS2 Amplitude", "channel_index"=0 ("y")) -> ()  [unwired: 9 in, 1 out]
          }
        }
      }
      frame "Read Voltage" {
        w211 = State."Exit"  # Next State
        w210 = State."Capture"  # Next State
        w218 = i8 0 ("channel")
        w231 = FALSE  # Stop Loop?
        n86 = Unbundle By Name(w212) -> ("Numeric <Replace Me>"=w227:dbl)
        n87 = Multiply(x=w227, y=1024) -> (x*y=w219:dbl)
        n88 = call "Read Voltage Datas.vi"("length"=w219, "channel"=i8 0) -> ("error out"=w215:errorcluster, "buffer out"=w216:dbl[], "function return"=→"ReadVoltageData Return":u32)  [unwired: 7 in]
        n89 = call "Read Voltage Datas.vi"("error in (no error)"=w215, "length"=w219, "channel"=i8 1) -> ("error out"=w214:errorcluster, "buffer out"=w223:dbl[])  [unwired: 6 in, 1 out]
        n90 = call "Read Voltage Datas.vi"("error in (no error)"=w214, "length"=w219, "channel"=i8 2) -> ("error out"=w213:errorcluster, "buffer out"=w222:dbl[])  [unwired: 6 in, 1 out]
        n91 = call "Read Voltage Datas.vi"("error in (no error)"=w213, "length"=w219, "channel"=i8 3) -> ("buffer out"=w221:dbl[])  [unwired: 6 in, 2 out]
        n92 = Unbundle By Name(w212) -> ("Boolean <Is Exit>"=w208:bool)
        n93 = Build Array(w216, w223, w222, w221) -> (w220:dbl[][])
        n94 = Array Subset(array=w220, index (row)=w218, length (row)=w219, index (col)=w218, length (col)=w219) -> (→"Voltage Wave":dbl[][])
        n95 = Select(t=w211, s=w208, f=w210) -> (s? t:f=w209:T2)
      }
      frame "Read IO" {
        w233 = FALSE  # Stop Loop?
        w234 = State."Wait for Event"  # Next State
        w240 = 16 ("front")
        w237 = 1 ("front")
        n96 = call "Get IO In State.vi"() -> ("function return"=w236:u32)  [unwired: 10 in, 1 out]
        "IO Read Return" <- w236
        n97 = And(x=w236, y=w240) -> (x .and. y?=w239:u32)
        n98 = And(x=w236, y=w237) -> (x .and. y?=w235:u32)
        n99 = Equal?(x=w235, y=w237) -> (x = y?=→"IO0":bool)
        n100 = Equal?(x=w239, y=w240) -> (x = y?=→"IO4":bool)
      }
      frame "Exit" {
        w246 = TRUE  # Stop Loop?
        w248 = State."Exit"  # (Value Not Used)
        # "#CodeNeeded - Add any required cleanup code here."
        # "The state value is not used here since this is the last iteration of the state machine loop."
        # "Exit - Exit the application."
        n101 = flat-sequence {
          tunnel: [w250] -> w244
          tunnel: w244 -> [w257]
          frame #0 {
            w251 = i8 16  # IO Num
            w250 = i8 0  # en
            n102 = for {
              N: w251 -> [_]
              tunnel: w250 -> [w254]
              i -> [w255]
              n103 = feedback #1() -> (w252:errorcluster)  [unwired: 1 in]
              n104 = call "IO Enable.vi"("error in (no error)"=w252, "enable"=w254, "channel"=w255) -> ("error out"=w253:errorcluster)  [unwired: 8 in]
              n105 = feedback-in #1(w253) -> ()
            }
            n106 = Wait (ms)(milliseconds to wait=1000) -> ()  [unwired: 1 out]
          }
          frame #1 {
            w259 = i8 1  # channel
            w258 = i8 0  # channel
            n107 = call "DDS Output Enable.vi"("enable"=w257, "channel_index"=w258) -> ("error out"=w260:errorcluster)  [unwired: 9 in]
            n108 = call "DDS Output Enable.vi"("error in (no error)"=w260, "enable"=w257, "channel_index"=w259) -> ()  [unwired: 8 in, 1 out]
            n109 = Wait (ms)(milliseconds to wait=1000) -> ()  [unwired: 1 out]
          }
          frame #2 {
            n110 = call "Finish Dll.vi"() -> ()  [unwired: 10 in, 2 out]
          }
        }
      }
    }
    n111 = Or(x=w7, y=w6) -> (x .or. y?=w8:bool)
  }
  n112 = call <vilib>:"Simple Error Handler.vi"("error in (no error)"=w2) -> ("error out"=w1:errorcluster)  [unwired: 4 in, 4 out]
  n113 = disable-structure shown="RUN_TIME_ENGINE==True" {
    disable-tunnel: w1 -> [_ _]
    frame condition #0 (active) {
    }
    frame condition #1 {
      # "Call Quit LabVIEW if running as a built application."
      n114 = Quit LabVIEW() -> ()  [unwired: 1 in]
    }
  }
